vi "arduino 1.vi"() -> ()   [LabVIEW 2018]
uses:
  <vilib>/Instr/_visa.llb/VISA Configure Serial Port (Instr).vi
panel:
  out "Blinking":bool
  out "VISA resource name out":refnum<visa-resource-name>
  out "read buffer":string
  in  "stop":bool
  in  "VISA resource name":refnum<visa-resource-name>
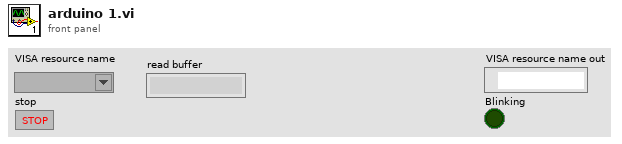
[diagram p1: front panel]
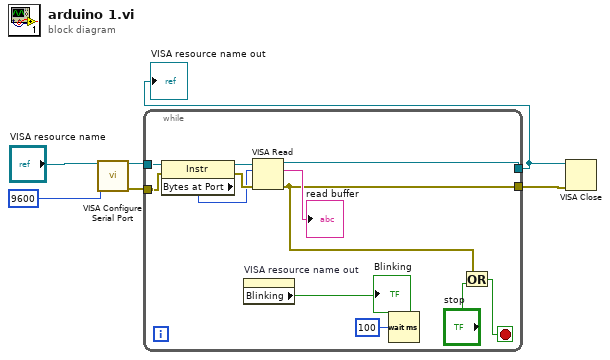
[diagram p0: block diagram]
diagram:
  n1 = call-poly "VISA Configure Serial Port"("VISA resource name"="VISA resource name", "baud rate (9600)"=u32 9600) -> ("VISA resource name out"=w4:refnum<visa-resource-name>, "error out"=w3:errorcluster)  [unwired: 12 in]
  n2 = while {
    tunnel: w4 -> [w12]
    tunnel: [w18] -> w1
    tunnel: w3 -> [w11]
    tunnel: [w13] -> w2
    stop <- w15 stop-if-true
    n3 = property class="Instr"(reference=w12, error in=w11) -> (reference out=w8:refnum<visa-resource-name>, error out=w10:errorcluster, "Bytes at Port"=w9:u32)
    n4 = property on="VISA resource name out" class="VISAName"() -> ("Blinking"=→"Blinking":bool)  [unwired: 2 in, 2 out]
    n5 = VISA Read(VISA resource name=w8, byte count=w9, error in (no error)=w10) -> (VISA resource name out=w18:refnum<visa-resource-name>, read buffer=→"read buffer":string, error out=w13:errorcluster)  [unwired: 1 out]
    n6 = Wait (ms)(milliseconds to wait=u32 100) -> ()  [unwired: 1 out]
    n7 = Or(x=w13, y="stop") -> (x .or. y?=w15:bool)
  }
  "VISA resource name out" <- w1
  n8 = VISA Close(VISA resource name=w1, error in (no error)=w2) -> ()  [unwired: 1 out]
